vi "net.vi"() -> ()   [LabVIEW 2021]
uses:
  <vilib>/Analysis/4window.llb/Flat Top Window (DBL).vi
  <vilib>/Analysis/2dsp.llb/Real FFT.vi
  <vilib>/Analysis/4window.llb/AllCosWindow (DBL).vi
  <vilib>/Waveform/WDTOps.llb/WDT Index Channel DBL.vi
  <vilib>/Waveform/WDTOps.llb/WDT Get Waveform Subset DBL.vi
  <vilib>/Analysis/3filter.llb/Butterworth Filter (DBL).vi
  <vilib>/Analysis/NI_AALPro.lvlib
  <vilib>/Analysis/NI_AALBase.lvlib
panel:
  out "widmo gloski po filtracji":waveform(dbl)(graph)
  out "gloska po filtracji":dbl[](graph)
  out "widmo czestotliwosciowe głoski":waveform(dbl)(graph)
  out "Głoska":dbl[](graph)
  out "f probk. [Hz]":dbl
  out "N":dbl
  out "Całkowity sygnał":waveform(dbl)[](graph)
  in  "Path":path
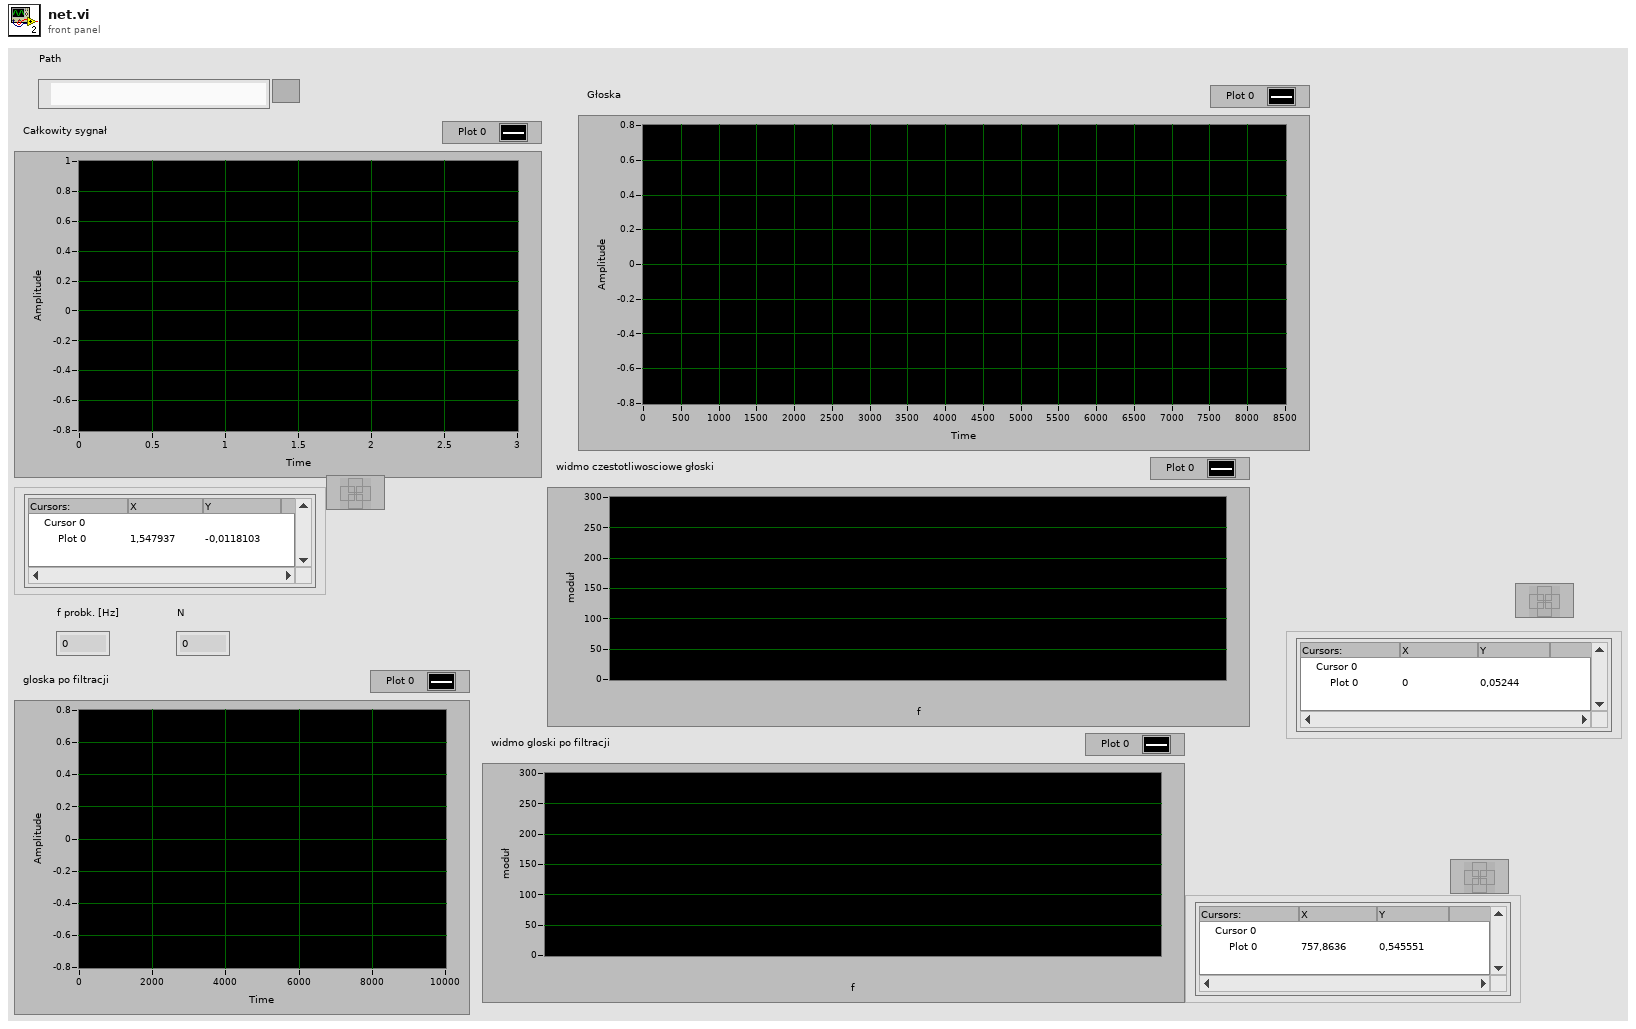
[diagram p1: front panel]
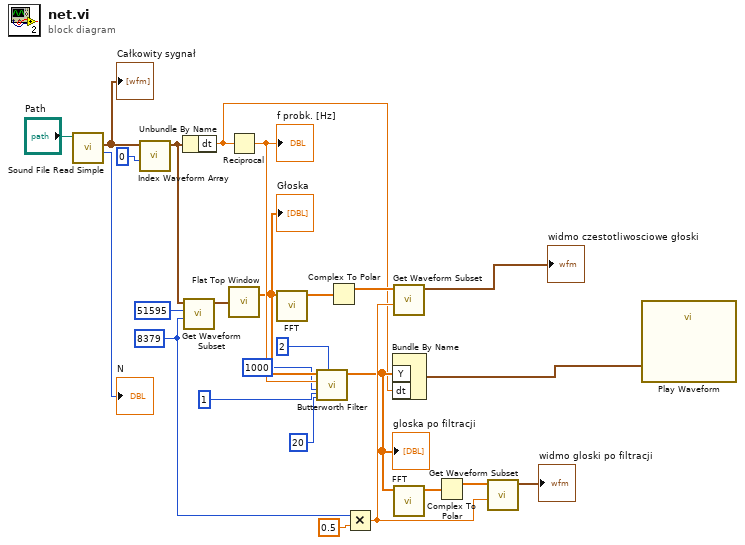
[diagram p0: block diagram]
diagram:
  w16 = 8379
  n1 = call <vilib>:"Sound File Read Simple.vi"("path"="Path") -> ("offset"=→"N":i32, "data"=w23:waveform(dbl)[])  [unwired: 7 in, 2 out]
  "Całkowity sygnał" <- w23
  n2 = call-poly <vilib>:"Index Waveform Array.vi"("index"=0, "waveform array"=w23) -> ("waveform"=w21:waveform(dbl))  [unwired: 8 in, 1 out]
  n3 = Unbundle By Name(w21) -> ("dt"=w4:dbl)
  n4 = call-poly <vilib>:"Get Waveform Subset.vi"("duration"=w16, "start samples/time"=51595, "waveform in"=w21) -> ("waveform out"=w3:waveform(dbl))  [unwired: 3 in, 3 out]
  n5 = Reciprocal(x=w4) -> (1/x=w6:dbl)
  "f probk. [Hz]" <- w6
  n6 = call-poly <vilib>:"Flat Top Window.vi"("X"=w3) -> ("Windowed X"=w2:dbl[])  [unwired: 1 out]
  "Głoska" <- w2
  n7 = call-poly <vilib>:"FFT.vi"("X"=w2) -> ("FFT {X}"=w19:cdb[])  [unwired: 9 in, 1 out]
  n8 = call-poly <vilib>:"Butterworth Filter.vi"("order"=1, "filter type"=2, "low cutoff freq: fl"=20, "high cutoff freq: fh"=1000, "sampling freq: fs"=w6, "X"=w2) -> ("Filtered X"=w7:dbl[])  [unwired: 2 in, 1 out]
  "gloska po filtracji" <- w7
  n9 = Complex To Polar(r * e^(i*theta)=w19) -> (r=w18:dbl[])  [unwired: 1 out]
  n10 = Multiply(x=w16, y=0.5) -> (x*y=w10:dbl)
  n11 = Bundle By Name("Y"=w7, "dt"=w4) -> (w5:waveform(dbl))  [unwired: 1 in]
  n12 = call-poly <vilib>:"Get Waveform Subset.vi"("duration"=w10, "waveform in"=w18) -> ("waveform out"=→"widmo czestotliwosciowe głoski":waveform(dbl))  [unwired: 4 in, 3 out]
  n13 = call-poly <vilib>:"FFT.vi"("X"=w7) -> ("FFT {X}"=w13:cdb[])  [unwired: 9 in, 1 out]
  n14 = Complex To Polar(r * e^(i*theta)=w13) -> (r=w12:dbl[])  [unwired: 1 out]
  n15 = call-poly <vilib>:"Get Waveform Subset.vi"("duration"=w10, "waveform in"=w12) -> ("waveform out"=→"widmo gloski po filtracji":waveform(dbl))  [unwired: 4 in, 3 out]
  n16 = call "Play Waveform"("Data"=w5) -> ()  [unwired: 18 in, 1 out]
